vi "Run All Tests.vi"(8 "error in (no error)":errorcluster, 11 "Execution UI In":refnum<class "Execution UI.lvclass">) -> (0 "error out":errorcluster, 3 "Execution UI Out":refnum<class "Execution UI.lvclass">)   [LabVIEW 2020, in "Execution UI.lvclass"]
uses:
  Execution UI.lvclass
  Execution UI.lvclass/Execution UI.ctl
  Helper Classes/Result Table/Result Table/Result Table.lvclass/Result Table.ctl
  Helper Classes/Test Finder/Test Finder.lvclass
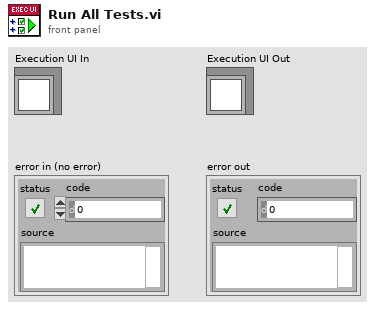
[diagram p1: front panel]
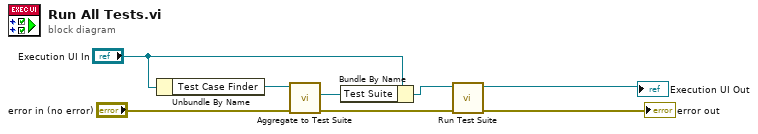
[diagram p0: block diagram]
diagram:
  n1 = Unbundle By Name("Execution UI In") -> ("Test Case Finder"=w5:refnum<class "Test Finder.lvclass">)
  n2 = call "Aggregate to Test Suite.vi"("error in (no error)"="error in (no error)", "Test Finder In"=w5) -> ("error out"=w2:errorcluster, "Test Suite"=w3:refnum<class "LUnit Test Suite.lvclass">)  [unwired: 7 in, 1 out]
  n3 = Bundle By Name(cluster="Execution UI In", "Test Suite"=w3) -> (w4:refnum<class "Execution UI.lvclass">)
  n4 = call "Run Test Suite.vi"("error in (no error)"=w2, "Execution UI In"=w4) -> ("error out"=→"error out":errorcluster, "Execution UI Out"=→"Execution UI Out":refnum<class "Execution UI.lvclass">)  [unwired: 8 in]
